vi "Memory Buffer.vi"(8 "error in (no error)":errorcluster, 9 "Dim Value (1)":i16=1 min=1 max=128 step=1, 10 "Memory Mode (0: Dim)":u32(slide) max=3 step=1, 11 "VISA resource name":refnum<visa-resource-name>) -> (0 "error out":errorcluster, 3 "VISA resource name out":refnum<visa-resource-name>)   [LabVIEW 2015, in "Agilent 428X Series.lvlib"]
doc: "This function controls the HP 428XA's data buffer."
uses:
  Agilent 428X Series.lvlib
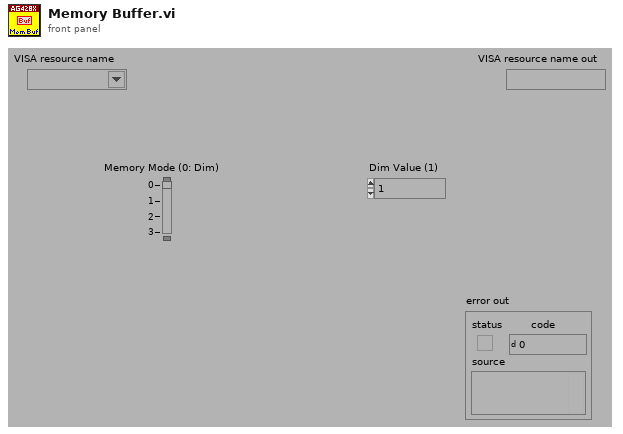
[diagram p1: front panel]
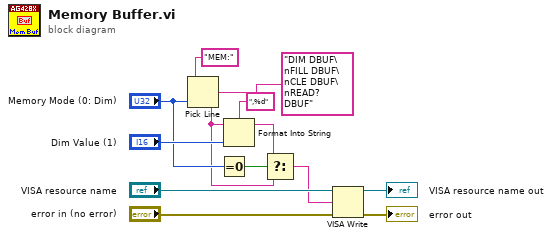
[diagram p0: block diagram]
diagram:
  n1 = Pick Line(string ("")="MEM:", multi-line string="DIM DBUF\nFILL DBUF\nCLE DBUF\nREAD? DBUF", line index="Memory Mode (0: Dim)") -> (output string=w2:string)
  n2 = Equal To 0?(x="Memory Mode (0: Dim)") -> (x = 0?=w4:bool)
  n3 = Format Into String(format string=",%d", initial string=w2, "Dim Value (1)") -> (resulting string=w3:string)  [unwired: 1 in, 1 out]
  n4 = Select(t=w3, s=w4, f=w2) -> (s? t:f=w1:string)
  n5 = VISA Write(VISA resource name="VISA resource name", write buffer=w1, error in (no error)="error in (no error)") -> (VISA resource name out=→"VISA resource name out":refnum<visa-resource-name>, error out=→"error out":errorcluster)  [unwired: 1 out]
